vi "ctl -- name dispatcher.vi"(8 "sweep folder path":path, 11 "ctl name dispatch":T1) -> (0 "file path":path, 1 "file or folder exists?":bool, 3 "ctl file name":string)   [LabVIEW 2015]
uses:
  ctl -- name dispatcher -- action.ctl
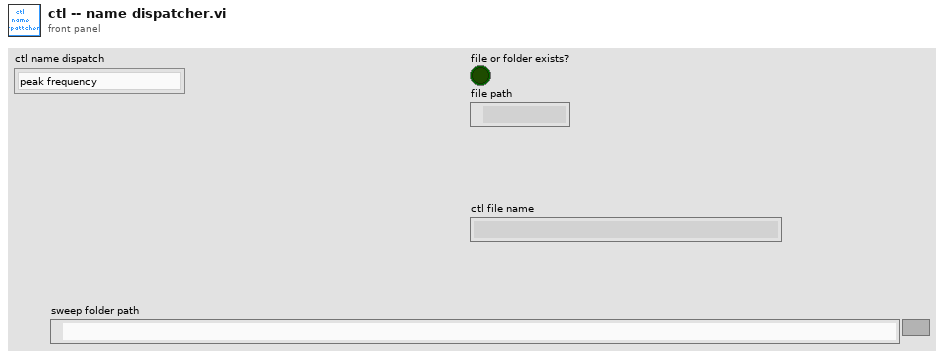
[diagram p1: front panel]
types:
  T1 = typedef "ctl -- name dispatcher -- action.ctl" = enum16{"peak frequency", "peak frequency DUMP", "peak gamma DUMP", "peak gamma", "peak frequency TEST", "peak gamma TEST", "ultrasonic power", "time in gamma", "set temperature ", "set temperature timer", "peak default gamma", "last scan file", "peak freq gamma TEST", "peak NAMES", "errors", "P_I_D", "P", "I", "D", "power vs time", "power vs time TIMER", "void", "power log", "set temperature - SINE", "itc ltc log", "peak - time in gamma"}
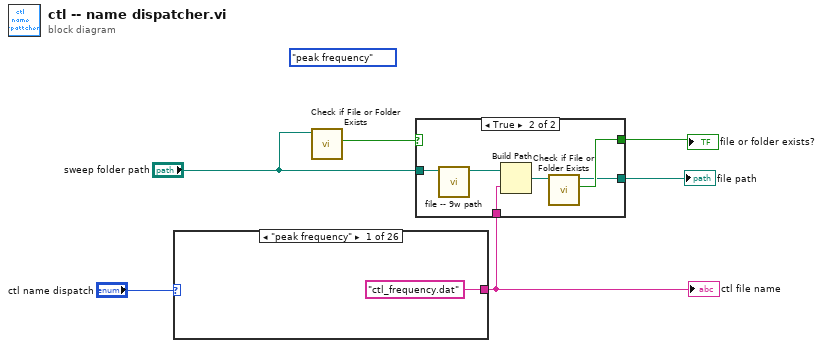
[diagram p0: block diagram]
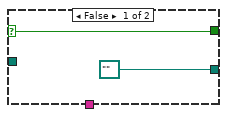
[diagram p2: hidden frame]
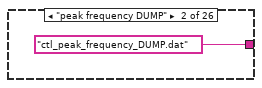
[diagram p3: hidden frame]
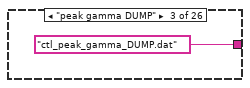
[diagram p4: hidden frame]
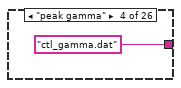
[diagram p5: hidden frame]
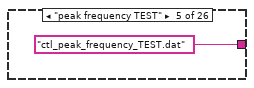
[diagram p6: hidden frame]
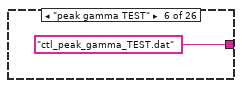
[diagram p7: hidden frame]
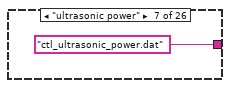
[diagram p8: hidden frame]
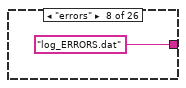
[diagram p9: hidden frame]
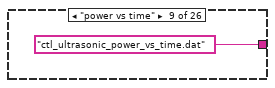
[diagram p10: hidden frame]
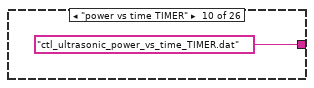
[diagram p11: hidden frame]
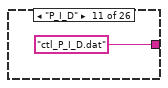
[diagram p12: hidden frame]
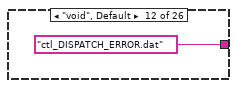
[diagram p13: hidden frame]
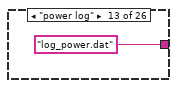
[diagram p14: hidden frame]
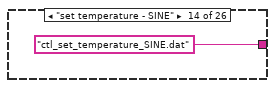
[diagram p15: hidden frame]
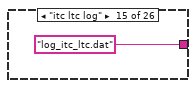
[diagram p16: hidden frame]
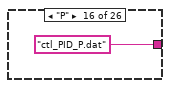
[diagram p17: hidden frame]
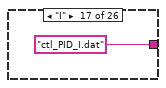
[diagram p18: hidden frame]
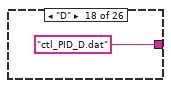
[diagram p19: hidden frame]
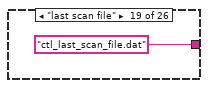
[diagram p20: hidden frame]
diagram:
  (unwired) ctl_--_name_dispatcher_--_action."peak frequency" ("ctl name dispatch")
  n1 = case shown="\"peak frequency\"" "ctl name dispatch" {
    tunnel: ["ctl_frequency.dat" ("freq PID file") "ctl_peak_frequency_DUMP.dat" ("freq PID file") "ctl_peak_gamma_DUMP.dat" ("freq PID file") "ctl_gamma.dat" ("freq PID file") "ctl_peak_frequency_TEST.dat" ("freq PID file") "ctl_peak_gamma_TEST.dat" ("freq PID file") "ctl_ultrasonic_power.dat" ("freq PID file") "log_ERRORS.dat" ("freq PID file") "ctl_ultrasonic_power_vs_time.dat" ("freq PID file") "ctl_ultrasonic_power_vs_time_TIMER.dat" ("freq PID file") "ctl_P_I_D.dat" ("freq PID file") "ctl_DISPATCH_ERROR.dat" ("freq PID file") "log_power.dat" ("freq PID file") "ctl_set_temperature_SINE.dat" ("freq PID file") "log_itc_ltc.dat" ("freq PID file") "ctl_PID_P.dat" ("freq PID file") "ctl_PID_I.dat" ("freq PID file") "ctl_PID_D.dat" ("freq PID file") "ctl_last_scan_file.dat" ("freq PID file") "ctl_peak_freq_gamma_TEST.dat" ("freq PID file") "ctl_peak_NAMES.dat" ("freq PID file") "ctl_time_in_gamma.dat" ("freq PID file") "ctl_peak_time_in_gamma.dat" ("freq PID file") "ctl_set_temperature.dat" ("freq PID file") "ctl_set_temperature_TIMER.dat" ("freq PID file") "ctl_peak_default_gamma.dat" ("freq PID file")] -> w6
    frame "peak frequency" {
    }
    frame "peak frequency DUMP" {
    }
    frame "peak gamma DUMP" {
    }
    frame "peak gamma" {
    }
    frame "peak frequency TEST" {
    }
    frame "peak gamma TEST" {
    }
    frame "ultrasonic power" {
    }
    frame "errors" {
    }
    frame "power vs time" {
    }
    frame "power vs time TIMER" {
    }
    frame "P_I_D" {
    }
    frame "void", Default {
    }
    frame "power log" {
    }
    frame "set temperature - SINE" {
    }
    frame "itc ltc log" {
    }
    frame "P" {
    }
    frame "I" {
    }
    frame "D" {
    }
    frame "last scan file" {
    }
    frame "peak freq gamma TEST" {
    }
    frame "peak NAMES" {
    }
    frame "time in gamma" {
    }
    frame "peak - time in gamma" {
    }
    frame "set temperature " {
    }
    frame "set temperature timer" {
    }
    frame "peak default gamma" {
    }
  }
  "ctl file name" <- w6
  n2 = call <vilib>:"Check if File or Folder Exists.vi"("path"="sweep folder path") -> ("file or folder exists?"=w4:bool)  [unwired: 8 in, 2 out]
  n3 = case shown="True" w4 {
    selector: w4 -> [w34 _]
    tunnel: w6 -> [_ w38]
    tunnel: "sweep folder path" -> [_ w37]
    tunnel: [w34 w36] -> w3
    tunnel: [path "" ("dup path") w35] -> w2
    frame False {
    }
    frame True {
      n4 = call "file -- 9w path.vi"("sweep folder"=w37) -> ("9w path"=w40:path)  [unwired: 10 in]
      n5 = Build Path(base path=w40, name or relative path=w38) -> (appended path=w39:path)
      n6 = call <vilib>:"Check if File or Folder Exists.vi"("path"=w39) -> ("file or folder exists?"=w36:bool, "dup path"=w35:path)  [unwired: 8 in, 1 out]
    }
  }
  "file or folder exists?" <- w3
  "file path" <- w2
